vi "GlobalVariables.vi"() -> ()   [LabVIEW 2020]
panel:
  out "HistogramEnabled":bool
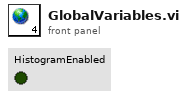
[diagram p1: front panel]
diagram:
